vi "Base64 Encode.vi"(10 "error in (no error)":errorcluster, 11 "String":string) -> (2 "error out":errorcluster, 3 "Encoded String":string)   [LabVIEW 2018]
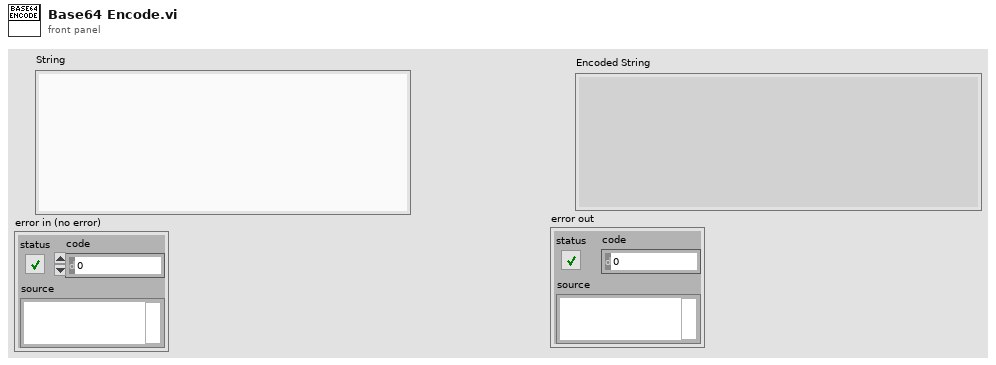
[diagram p1: front panel]
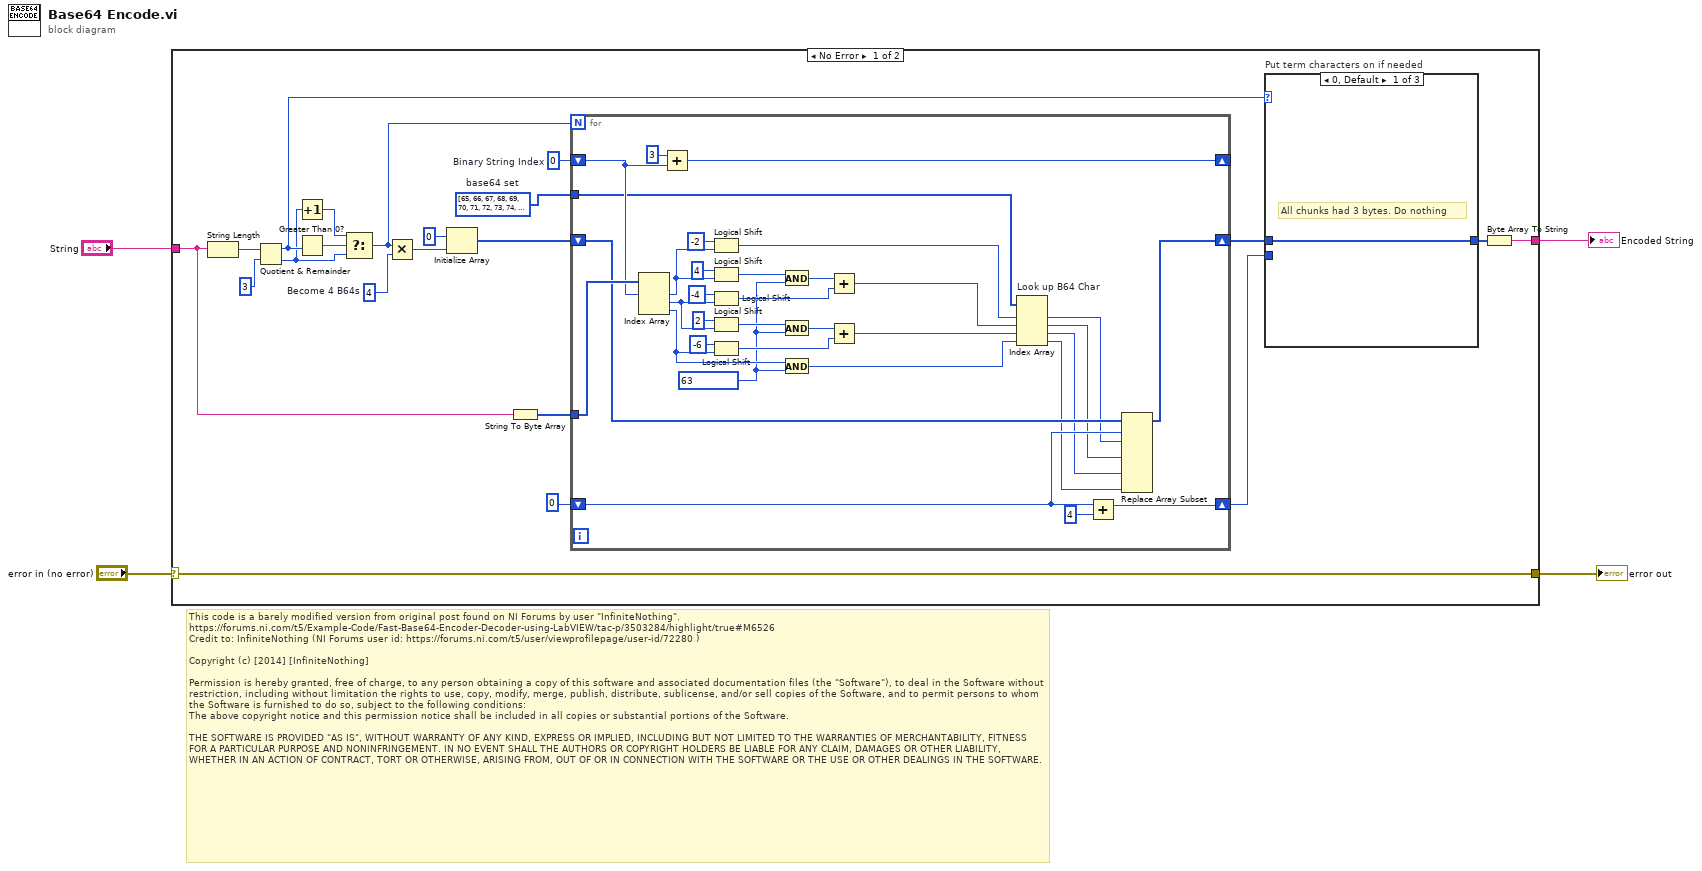
[diagram p0: block diagram]
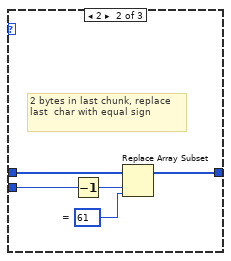
[diagram p2: hidden frame]
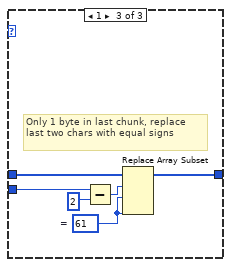
[diagram p3: hidden frame]
diagram:
  # "This code is a barely modified version from original post found on NI Forums by user \"InfiniteNothing\".\nhttps://forums.ni.com/t5/Example-Code/Fast-Base64-Encoder-Decoder-using-LabVIEW/tac-p/3503284/highlight/true#M6526\nCredit to: InfiniteNothing (NI Forums user id: https://forums.ni.com/t5/user/viewprofilepage/user-id/72280 )\n\nCopyright (c) [2014] [InfiniteNothing]\n\nPermission is hereby granted, free of charge, to any person obtaining a copy of this software and associated documentation files (the \"Software\"), to deal in the Software without restriction, including without limitation the rights to use, copy, modify, merge, publish, distribute, sublicense, and/or sell copies of the Software, and to permit persons to whom the Software is furnished to do so, subject to the following conditions:\nThe above copyright notice and this permission notice shall be included in all copies or substantial portions of the Software.\n\nTHE SOFTWARE IS PROVIDED \"AS IS\", WITHOUT WARRANTY OF ANY KIND, EXPRESS OR IMPLIED, INCLUDING BUT NOT LIMITED TO THE WARRANTIES OF MERCHANTABILITY, FITNESS FOR A PARTICULAR PURPOSE AND NONINFRINGEMENT. IN NO EVENT SHALL THE AUTHORS OR COPYRIGHT HOLDERS BE LIABLE FOR ANY CLAIM, DAMAGES OR OTHER LIABILITY, WHETHER IN AN ACTION OF CONTRACT, TORT OR OTHERWISE, ARISING FROM, OUT OF OR IN CONNECTION WITH THE SOFTWARE OR THE USE OR OTHER DEALINGS IN THE SOFTWARE."
  n1 = case shown="No Error" "error in (no error)" {
    selector: "error in (no error)" -> [w7 w71]
    tunnel: "String" -> [w8 _]
    tunnel: [w6 _] -> w3
    tunnel: [w7 w71] -> w1
    frame No Error {
      w5 = u8[] [65, 66, 67, 68, 69, 70, 71, 72, 73, 74, 75, 76, 77, 78, 79, 80, 81, 82, 83, 84, 85, 86, 87, 88, 89, 90, 97, 98, 99, 100, 101, 102, 103, 104, 105, 106, 107, 108, 109, 110, 111, 112, 113, 114, 115, 116, 117, 118, 119, 120, 121, 122, 48, 49, 50, 51, 52, 53, 54, 55, 56, 57, 43, 47]  # base64 set
      w13 = 4  # Become 4 B64s
      w17 = 0  # Binary String Index
      n2 = String Length(string=w8) -> (length=w24:i32)
      n3 = Quotient & Remainder(x=w24, y=3 ("Chunks of 3 U8s")) -> (x-y*floor(x/y)=w22:i32, floor(x/y)=w20:i32)
      n4 = Increment(x=w20) -> (x+1=w19:i32)
      n5 = Greater Than 0?(x=w22) -> (x > 0?=w21:bool)
      n6 = Select(t=w19, s=w21, f=w20) -> (s? t:f=w15:i32)
      n7 = Multiply(x=w15, y=w13) -> (x*y=w14:i32)
      n8 = Initialize Array(u8 0 ("element"), w14) -> (w11:u8[])
      n9 = String To Byte Array(string=w8) -> (unsigned byte array=w10:u8[])
      n10 = for {
        N: w15 -> [_]
        tunnel: w10 -> [w70]
        shift-right: [w68] -> _
        shift-left: w17 -> [w69]
        shift-right: [w65] -> w25
        shift-left: 0 ("B64 String Index") -> [w51]
        shift-right: [w52] -> w9
        shift-left: w11 -> [w53]
        tunnel: w5 -> [w38]
        w39 = u8 63 ("y")
        n11 = Index Array(array=w70, index #1=w69) -> (element #1=w63:u8, element #2=w58:u8, element #3=w55:u8)  [unwired: 2 in]
        n12 = Add(x=3 ("Chunks of 3 U8s"), y=w69) -> (x+y=w68:i32)
        n13 = Logical Shift(y=i8 -2, x=w63) -> (x << y=w64:u8)
        n14 = Logical Shift(y=i8 4, x=w63) -> (x << y=w46:u8)
        n15 = Logical Shift(y=i8 -4, x=w58) -> (x << y=w60:u8)
        n16 = Logical Shift(y=i8 2, x=w58) -> (x << y=w43:u8)
        n17 = Logical Shift(y=i8 -6, x=w55) -> (x << y=w56:u8)
        n18 = And(x=w46, y=w39) -> (x .and. y?=w45:u8)
        n19 = And(x=w43, y=w39) -> (x .and. y?=w42:u8)
        n20 = And(x=w55, y=w39) -> (x .and. y?=w54:u8)
        n21 = Add(x=w45, y=w60) -> (x+y=w44:u8)
        n22 = Add(x=w42, y=w56) -> (x+y=w41:u8)
        n23 = Index Array "Look up B64 Char"(array=w38, index #1=w64, index #2=w44, index #3=w41, index #4=w54) -> (element #1=w50:u8, element #2=w49:u8, element #3=w48:u8, element #4=w47:u8)
        n24 = Add(x=w51, y=4 ("Become 4 B64s")) -> (x+y=w65:i32)
        n25 = Replace Array Subset(array=w53, new element #1=w50, index #1=w51, new element #2=w49, new element #3=w48, new element #4=w47) -> (w52:u8[])  [unwired: 3 in]
      }
      n26 = case "Put term characters on if needed" shown="0, Default" w22 {
        tunnel: w9 -> [w26 w31 w37]
        tunnel: [w26 w30 w36] -> w23
        tunnel: w25 -> [_ w29 w34]
        frame 0, Default {
          # "All chunks had 3 bytes. Do nothing"
        }
        frame 2 {
          w27 = u8 61  # =
          # "2 bytes in last chunk, replace last  char with equal sign"
          n27 = Decrement(x=w29) -> (x-1=w28:i32)
          n28 = Replace Array Subset(array=w31, new element=w27, index=w28) -> (w30:u8[])
        }
        frame 1 {
          w32 = u8 61  # =
          # "Only 1 byte in last chunk, replace last two chars with equal signs"
          n29 = Subtract(x=w34, y=2) -> (x-y=w35:i32)
          n30 = Replace Array Subset(array=w37, new element #1=w32, index #1=w35, new element #2=w32) -> (w36:u8[])  [unwired: 1 in]
        }
      }
      n31 = Byte Array To String(unsigned byte array=w23) -> (string=w6:string)
    }
    frame Error {
    }
  }
  "Encoded String" <- w3
  "error out" <- w1
